vi "GT Get Axis Prf Vel.vi"(6 "pClock":u32, 7 "count":i16, 8 "error in (no error)":errorcluster caption="错误输入（无错误）", 9 "pValue":dbl[](array[numeric]), 10 "axis":i16, 11 "cardNum":i16) -> (0 "error out":errorcluster caption="错误输出", 1 "pValue out":dbl[](array[numeric]), 3 "function return":i16, 4 "pClock out":u32)   [LabVIEW 2014, in "gts.lvlib"]
doc: "GT_API GT_GetAxisPrfVel(short cardNum,short axis,double *pValue,short count=1,unsigned long *pClock=NULL);"
uses:
  gts.lvlib
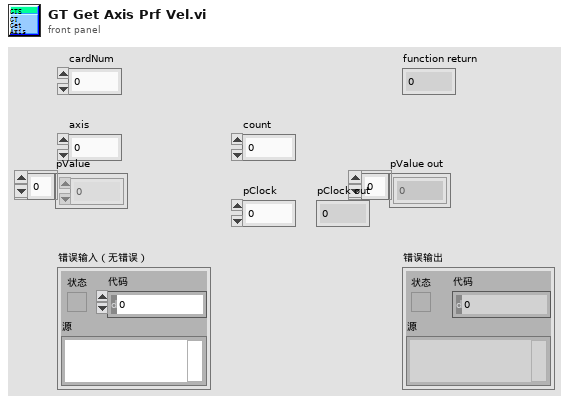
[diagram p1: front panel]
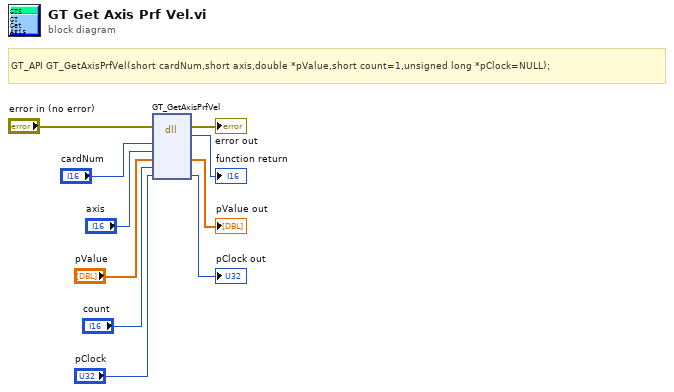
[diagram p0: block diagram]
diagram:
  # "GT_API GT_GetAxisPrfVel(short cardNum,short axis,double *pValue,short count=1,unsigned long *pClock=NULL);"
  n1 = dll-call lib="PTH2habs D固高科技资料GTS控制卡GTS卡18年上半年资料dllVC32bit\nmulti_cardgts.*" fn="GT_GetAxisPrfVel"(error in="error in (no error)", "cardNum"="cardNum", "axis"="axis", "pValue"="pValue", "count"="count", "pClock"="pClock") -> (error out=→"error out":errorcluster, "返回类型"=→"function return":i16, "pValue"=→"pValue out":dbl[], "pClock"=→"pClock out":u32)  [unwired: 5 in, 1 out]
